vi "tcsWEP_getEvent_detailedState.vi"(8 "error in (no error)":errorcluster, 11 "logevent_detailedState_Ctl":T1) -> (0 "error out":errorcluster, 2 "function return":i32, 3 "logevent_detailedState_Ctl out":T1)   [LabVIEW 2016, in "SALLV_tcsWEP.lvlib"]
doc: "int tcsWEP_shm_getEvent_detailedStateLV(tcsWEP_logevent_detailedStateLV *logevent_detailedState_Ctl );"
uses:
  SALLV_tcsWEP.lvlib
  DataTypes/logevent_detailedState.ctl
  SALLV_tcsWEP.so
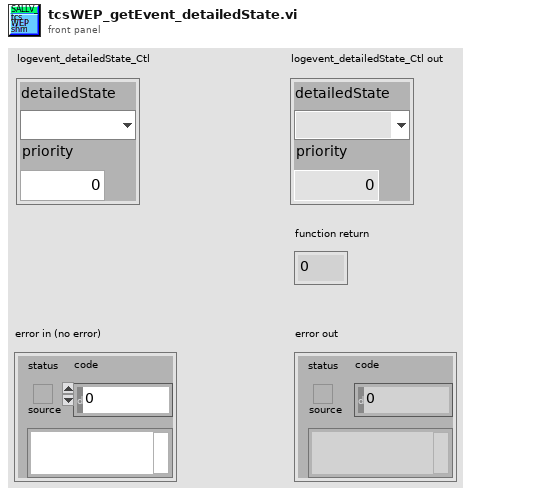
[diagram p1: front panel]
types:
  T1 = typedef "SALLV_tcsWEP.lvlib/logevent_detailedState.ctl" = cluster{"detailedState":enum32{"", "DisabledState", "EnabledState", "FaultState", "OfflineState", "StandbyState"}, "priority":i32}
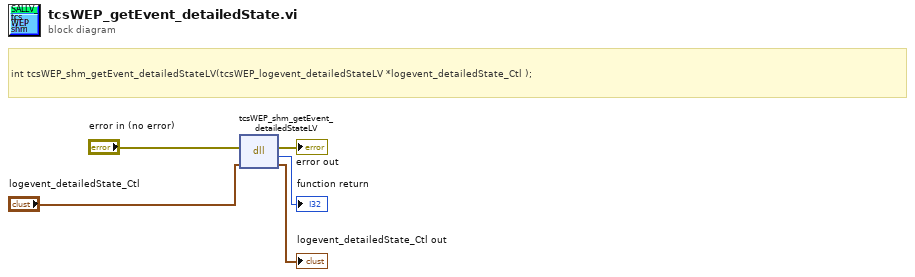
[diagram p0: block diagram]
diagram:
  # "int tcsWEP_shm_getEvent_detailedStateLV(tcsWEP_logevent_detailedStateLV *logevent_detailedState_Ctl );"
  n1 = dll-call lib="home/ttsai/Documents/salAPI/SALLV_tcsWEP.*" fn="tcsWEP_shm_getEvent_detailedStateLV"(error in="error in (no error)", "logevent_detailedState_Ctl"="logevent_detailedState_Ctl") -> (error out=→"error out":errorcluster, →"function return":i32, "logevent_detailedState_Ctl"=→"logevent_detailedState_Ctl out":T1)  [unwired: 2 in, 1 out]
